vi "Set Logging File Name.vi"(7 "error in":errorcluster, 9 "file name":string, 10 "logging section":T1=18446744073709551615 format="%.0x") -> (0 "error out":errorcluster, 3 "logging section out":T1 format="%.0x")   [LabVIEW 2020, in "AIM MIL-STD-1553 Scripting.lvlib"]
doc: "Specifies the name of the log file."
uses:
  AIM MIL-STD-1553 Scripting.lvlib
  <vilib>/NI VeriStand/Custom Device API/Custom Device Item Ref.ctl
  Constants.vi
  <vilib>/NI VeriStand/Custom Device API/Set Item Property (String).vi
  <vilib>/NI VeriStand/Custom Device API/Custom Device API.lvlib
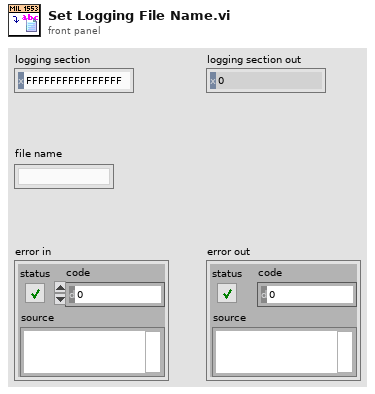
[diagram p1: front panel]
types:
  T1 = typedef "Custom Device API.lvlib/Custom Device Item Ref.ctl" = u64
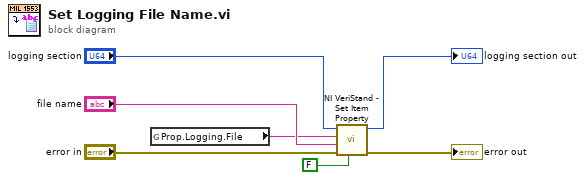
[diagram p0: block diagram]
diagram:
  n1 = global read "Constants.vi" "Prop.Logging.File"() -> (w1:string)
  n2 = call-poly <vilib>:"NI VeriStand - Set Item Property.vi"("Binary String (T)"=FALSE, "error in (no error)"="error in", "Value"="file name", "Property Name"=w1, "Item Ref in"="logging section") -> ("error out"=→"error out":errorcluster, "Item Ref out"=→"logging section out":T1)  [unwired: 4 in, 1 out]
